vi "Get Wire Type.vi"(8 "error in (no error)":errorcluster, 11 "I64 Wire in":refnum<class "LEN.lvclass">) -> (0 "error out":errorcluster, 2 "Wire Type":T1, 3 "I64 Wire out":refnum<class "LEN.lvclass">)   [LabVIEW 2020, in "Protobuf RAW.lvlib" / "LEN.lvclass"]
uses:
  LEN.lvclass
  Type Serializer/Wire Type.ctl
  Wire Type Group/Wire Type Group.lvclass
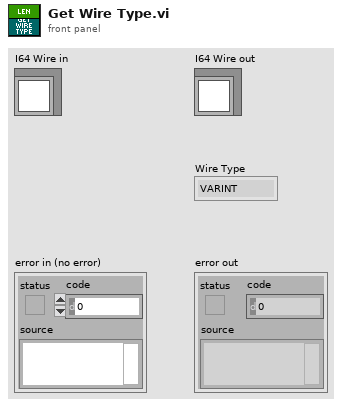
[diagram p1: front panel]
types:
  T1 = typedef "Protobuf RAW.lvlib/Wire Type Group.lvclass/Wire Type.ctl" = enum16{"VARINT", "I64", "LEN", "SGROUP", "EGROUP", "I32"}
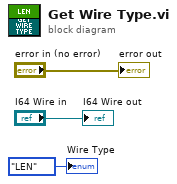
[diagram p0: block diagram]
diagram:
  "error out" <- "error in (no error)"
  "I64 Wire out" <- "I64 Wire in"
  "Wire Type" <- Wire_Type."LEN" ("Wire Type")
